vi "Preset_Edit_Res2txt.vi"(11 "Resolution":i32) -> (3 "Resolution text":string)   [LabVIEW 2020, in "Gviewer.lvclass"]
doc: "Convert resolution text"
uses:
  Gviewer.lvclass
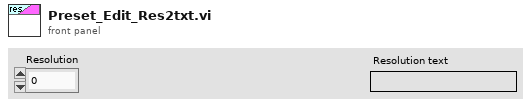
[diagram p1: front panel]
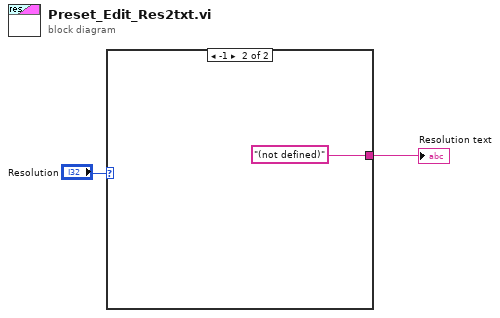
[diagram p0: block diagram]
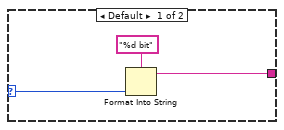
[diagram p2: hidden frame]
diagram:
  n1 = case shown="-1" "Resolution" {
    selector: "Resolution" -> [w5 _]
    tunnel: [w3 "(not defined)"] -> w1
    frame Default {
      n2 = Format Into String(format string="%d bit", w5) -> (resulting string=w3:string)  [unwired: 2 in, 1 out]
    }
    frame -1 {
    }
  }
  "Resolution text" <- w1
